vi "正弦波.vi"(9 "信号频率 Hz":dbl=1.0, 10 "采样点数 S":u32=1000 min=1000 max=1600000, 11 "采样率 [Hz]":dbl=1000.0 min=1000.0 max=1600000.0) -> (1 "Sine 波形 FXP":fxp<+/-,20,5>[](array[numeric]), 2 "Sine 波形":dbl[](array[numeric]))   [LabVIEW 2019]
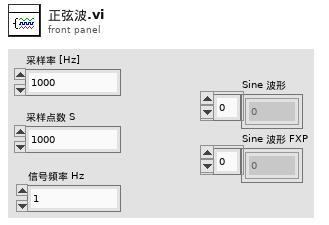
[diagram p1: front panel]
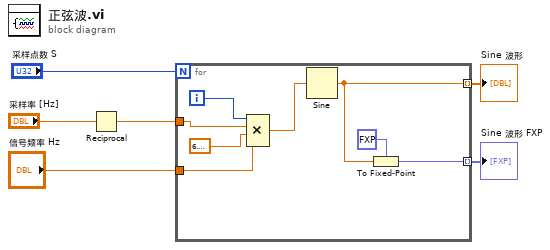
[diagram p0: block diagram]
diagram:
  n1 = Reciprocal(x="采样率 [Hz]") -> (1/x=w4:dbl)
  n2 = for {
    N: "采样点数 S" -> [_]
    tunnel: [w12] -> w2 mode=indexing
    tunnel: [w13] -> w1 mode=indexing
    tunnel: "信号频率 Hz" -> [w8]
    tunnel: w4 -> [w7]
    i -> [w10]
    n3 = Compound Arithmetic op=MULTIPLY ("复合运算")(w10, w7, 6.283185307179586, w8) -> (w9:dbl)
    n4 = Sine(x=w9) -> (sin(x)=w12:dbl)
    n5 = To Fixed-Point(fixed-point type=fxp<+/-,20,5> 0.0 ("定点类型"), number=w12) -> (fixed-point=w13:fxp<+/-,20,5>)
  }
  "Sine 波形" <- w2
  "Sine 波形 FXP" <- w1
